vi "Vector_Duplication.vi"(8 "error in (no error)":errorcluster, 10 "# duplicates":dbl=2.0, 11 "input vector":dbl[](array[numeric])=[1.0, 2.0, 3.0, 4.0, 5.0]) -> (0 "error out":errorcluster, 3 "Duplicated vector":dbl[](array[numeric]))   [LabVIEW 2023]
doc: "This VI duplicates a vector. The input vector will be reproduced a number which corresponds to the input # of duplicates.\nFor example, the input vector [123] will be [123123123] after a duplication of 3"
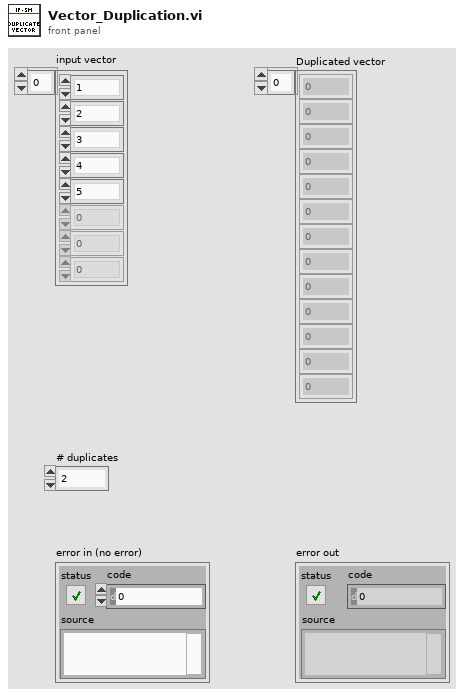
[diagram p1: front panel]
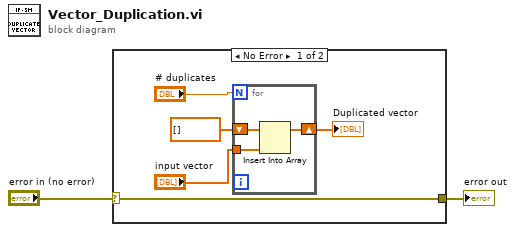
[diagram p0: block diagram]
diagram:
  n1 = case shown="No Error" "error in (no error)" {
    selector: "error in (no error)" -> [w5 w11]
    tunnel: [w5 w11] -> w1
    frame No Error {
      n2 = for {
        N: "# duplicates" -> [_]
        tunnel: "input vector" -> [w9]
        shift-right: [w8] -> w6
        shift-left: dbl[] [] -> [w10]
        n3 = Insert Into Array(array=w10, new element=w9) -> (w8:dbl[])  [unwired: 1 in]
      }
      "Duplicated vector" <- w6
    }
    frame Error {
    }
  }
  "error out" <- w1
